vi "HandleCollisions.vi"(8 "error in (no error)":errorcluster, 11 "Bouncer in":refnum<class "Bouncer.lvclass">) -> (0 "error out":errorcluster, 3 "Bouncer out":refnum<class "Bouncer.lvclass">)   [LabVIEW 2019, in "RT_Game.lvlib" / "Bouncer.lvclass"]
uses:
  Bouncer.lvclass
  C:/Users/FreshBob/Dropbox/VIs/myRIO_GameConsole/RT/RT_Game/Game/Game.lvclass
  PongBall/PongBall.lvclass
  C:/Users/FreshBob/Dropbox/VIs/myRIO_GameConsole/RT/RT_Game/GameObject/GameObject.lvclass
  PongPanel/PongPanel.lvclass
  Menu/States.ctl
  Game/Game.lvclass/Game.ctl
  Bouncer.lvclass/Bouncer.ctl
  BounceTarget/BounceTarget.lvclass
  Game/Read Player1Score.vi
  Game/Write Player1Score.vi
  Game/Read Player2Score.vi
  Game/Write Player2Score.vi
  Game/Read State.vi
  Game/Read Singleplayer.vi
  GameObject/GameObject.lvclass
  Game/Game.lvclass
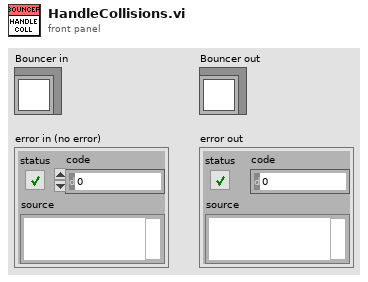
[diagram p1: front panel]
types:
  T1 = typedef "RT_Game.lvlib/Game.lvclass/States.ctl" = enum16{"Init", "Restart", "Menu", "Game", "Resume", "ToggleSingleplayer", "LoadNextGame", "ExitToMenu", "NewHighscore", "GameOver", "SlideOut"}
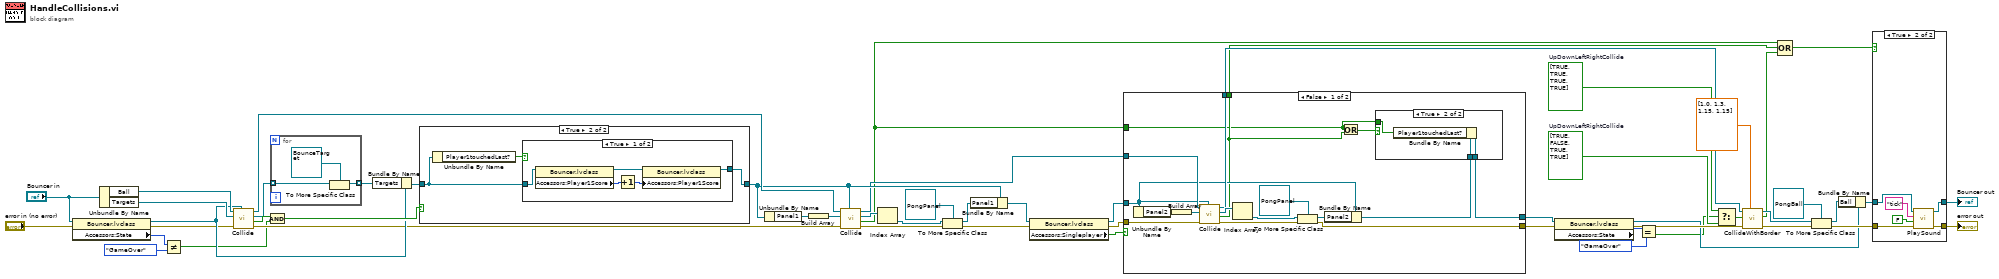
[diagram p0: block diagram]
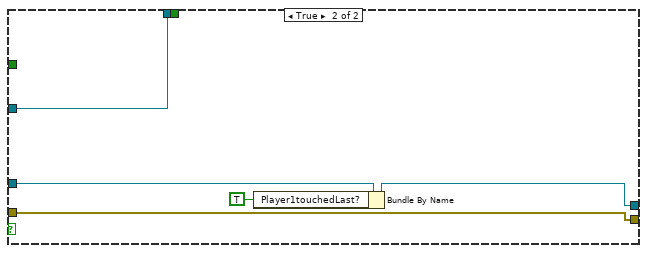
[diagram p3: hidden frame]
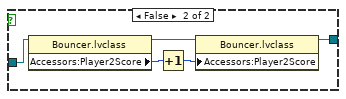
[diagram p6: hidden frame]
diagram:
  w27 = bool[] [TRUE, FALSE, TRUE, TRUE]  # UpDownLeftRightCollide
  w25 = bool[] [TRUE, TRUE, TRUE, TRUE]  # UpDownLeftRightCollide
  n1 = property class="Bouncer.lvclass"(reference="Bouncer in", error in="error in (no error)") -> (reference out=w35:refnum<class "Bouncer.lvclass">, error out=w34:errorcluster, "Accessors:State"=w6:T1)
  n2 = Unbundle By Name("Bouncer in") -> ("Ball"=w37:refnum<class "PongBall.lvclass">, "Targets"=w38:refnum<class "BounceTarget.lvclass">[])
  n3 = Not Equal?(x=w6, y=States."GameOver") -> (x != y?=w4:bool)
  n4 = call "Collide.vi"("RT_Game.lvlib:Game.lvclass"=w35, "error in (no error)"=w34, "Colliders"=w38, "Object in"=w37) -> ("error out"=w21:errorcluster, "collided"=w30:bool, "Colliders 2"=w23:refnum<class "GameObject.lvclass">[], "Object out"=w28:refnum<class "GameObject.lvclass">)  [unwired: 3 in, 1 out]
  n5 = for {
    tunnel: w23 -> [w56] mode=indexing
    tunnel: [w55] -> w53 mode=indexing
    n6 = To More Specific Class(target class=refnum<class "BounceTarget.lvclass"> refnum ("RT_Game.lvlib:BounceTarget.lvclass"), reference=w56) -> (specific class reference=w55:refnum<class "BounceTarget.lvclass">)  [unwired: 1 in, 1 out]
  }
  n7 = Compound Arithmetic op=AND(w30, w4) -> (w36:bool)
  n8 = Bundle By Name(cluster=w35, "Targets"=w53) -> (w52:refnum<class "Bouncer.lvclass">)
  n9 = case shown="True" w36 {
    tunnel: [w58 w61] -> w20
    tunnel: w52 -> [w58 w60]
    frame False {
    }
    frame True {
      n10 = Unbundle By Name(w60) -> ("Player1touchedLast?"=w59:bool)
      n11 = case shown="True" w59 {
        tunnel: [w64 w69] -> w61
        tunnel: w60 -> [w62 w67]
        frame True {
          n12 = property class="Bouncer.lvclass"(reference=w62) -> (reference out=w66:refnum<class "Bouncer.lvclass">, "Accessors:Player1Score"=w65:i32)  [unwired: 1 in, 1 out]
          n13 = Increment(x=w65) -> (x+1=w63:i32)
          n14 = property class="Bouncer.lvclass"(reference=w66, "Accessors:Player1Score"=w63) -> (reference out=w64:refnum<class "Bouncer.lvclass">)  [unwired: 1 in, 1 out]
        }
        frame False {
          n15 = property class="Bouncer.lvclass"(reference=w67) -> (reference out=w71:refnum<class "Bouncer.lvclass">, "Accessors:Player2Score"=w70:i32)  [unwired: 1 in, 1 out]
          n16 = Increment(x=w70) -> (x+1=w68:i32)
          n17 = property class="Bouncer.lvclass"(reference=w71, "Accessors:Player2Score"=w68) -> (reference out=w69:refnum<class "Bouncer.lvclass">)  [unwired: 1 in, 1 out]
        }
      }
    }
  }
  n18 = Unbundle By Name(w20) -> ("Panel1"=w51:refnum<class "PongPanel.lvclass">)
  n19 = Build Array(w51) -> (w29:refnum<class "PongPanel.lvclass">[])
  n20 = call "Collide.vi"("RT_Game.lvlib:Game.lvclass"=w20, "error in (no error)"=w21, "Colliders"=w29, "Object in"=w28) -> ("error out"=w47:errorcluster, "collided"=w12:bool, "Colliders 2"=w45:refnum<class "GameObject.lvclass">[], "Object out"=w18:refnum<class "GameObject.lvclass">)  [unwired: 3 in, 1 out]
  n21 = Index Array(array=w45) -> (element=w49:refnum<class "GameObject.lvclass">)  [unwired: 1 in]
  n22 = To More Specific Class(target class=refnum<class "PongPanel.lvclass"> refnum ("RT_Game.lvlib:PongPanel.lvclass"), reference=w49, error in=w47) -> (specific class reference=w50:refnum<class "PongPanel.lvclass">, error out=w48:errorcluster)
  n23 = Bundle By Name(cluster=w20, "Panel1"=w50) -> (w11:refnum<class "Bouncer.lvclass">)
  n24 = property class="Bouncer.lvclass"(reference=w11, error in=w48) -> (reference out=w10:refnum<class "Bouncer.lvclass">, error out=w8:errorcluster, "Accessors:Singleplayer"=w9:bool)
  n25 = case shown="False" w9 {
    tunnel: [w81 w97] -> w19
    tunnel: w18 -> [w80 w97]
    tunnel: w10 -> [w79 w96]
    tunnel: [w77 w94] -> w14
    tunnel: [w76 _] -> w13
    tunnel: w12 -> [w74 _]
    tunnel: w8 -> [w73 w95]
    tunnel: [w72 w95] -> w7
    frame False {
      n26 = Unbundle By Name(w79) -> ("Panel2"=w82:refnum<class "PongPanel.lvclass">)
      n27 = Build Array(w82) -> (w88:refnum<class "PongPanel.lvclass">[])
      n28 = call "Collide.vi"("RT_Game.lvlib:Game.lvclass"=w79, "error in (no error)"=w73, "Colliders"=w88, "Object in"=w80) -> ("error out"=w85:errorcluster, "collided"=w76:bool, "Colliders 2"=w87:refnum<class "GameObject.lvclass">[], "Object out"=w81:refnum<class "GameObject.lvclass">)  [unwired: 3 in, 1 out]
      n29 = Index Array(array=w87) -> (element=w84:refnum<class "GameObject.lvclass">)  [unwired: 1 in]
      n30 = To More Specific Class(target class=refnum<class "PongPanel.lvclass"> refnum ("RT_Game.lvlib:PongPanel.lvclass"), reference=w84, error in=w85) -> (specific class reference=w83:refnum<class "PongPanel.lvclass">, error out=w72:errorcluster)
      n31 = Bundle By Name(cluster=w79, "Panel2"=w83) -> (w78:refnum<class "Bouncer.lvclass">)
      n32 = Or(x=w74, y=w76) -> (x .or. y?=w75:bool)
      n33 = case shown="True" w75 {
        tunnel: w78 -> [w89 w92]
        tunnel: [w89 w91] -> w77
        tunnel: w74 -> [_ w90]
        frame False {
        }
        frame True {
          n34 = Bundle By Name(cluster=w92, "Player1touchedLast?"=w90) -> (w91:refnum<class "Bouncer.lvclass">)
        }
      }
    }
    frame True {
      n35 = Bundle By Name(cluster=w96, "Player1touchedLast?"=TRUE) -> (w94:refnum<class "Bouncer.lvclass">)
    }
  }
  n36 = property class="Bouncer.lvclass"(reference=w14, error in=w7) -> (reference out=w16:refnum<class "Bouncer.lvclass">, error out=w17:errorcluster, "Accessors:State"=w15:T1)
  n37 = Equal?(x=w15, y=States."GameOver" ("x")) -> (x = y?=w3:bool)
  n38 = Select(t=w25, s=w3, f=w27) -> (s? t:f=w26:bool[])
  n39 = call "CollideWithBorder.vi"("UpDownLeftRightBounce"=dbl[] [1.0, 1.3, 1.15, 1.15], "error in (no error)"=w17, "UpDownLeftRightCollide"=w26, "Object in"=w19) -> ("error out"=w39:errorcluster, "collided?"=w32:bool, "Object out"=w41:refnum<class "GameObject.lvclass">)  [unwired: 5 in]
  n40 = Compound Arithmetic op=OR(w12, w13, w32) -> (w33:bool)
  n41 = To More Specific Class(target class=refnum<class "PongBall.lvclass"> refnum ("Ball"), reference=w41, error in=w39) -> (specific class reference=w42:refnum<class "PongBall.lvclass">, error out=w43:errorcluster)
  n42 = Bundle By Name(cluster=w16, "Ball"=w42) -> (w40:refnum<class "Bouncer.lvclass">)
  n43 = case shown="True" w33 {
    tunnel: w43 -> [w98 w105]
    tunnel: [w98 w104] -> w44
    tunnel: w40 -> [w99 w103]
    tunnel: [w99 w102] -> w31
    frame False {
    }
    frame True {
      n44 = call "PlaySound.vi"("error in (no error)"=w105, "Overwrite"=FALSE, "Name"="tick", "Game in"=w103) -> ("error out"=w104:errorcluster, "Game out"=w102:refnum<class "Bouncer.lvclass">)  [unwired: 6 in]
    }
  }
  "error out" <- w44
  "Bouncer out" <- w31
